vi "NFL_Setpoint_Control.vi"(8 "error in":errorcluster, 9 "3 JSA60 DX812 XQ75":dbl, 10 "3 JSA60 DX811 XQ75":dbl, 11 "SI750.lvclass in":refnum<class "SI750.lvclass">) -> (0 "error out":errorcluster, 1 "NFL Setp Grad":dbl, 2 "NFL Setpoint":dbl, 3 "SI750.lvclass out":refnum<class "SI750.lvclass">)   [LabVIEW 2022 SP3, in "SI750.lvclass"]
uses:
  SI750.lvclass
  SI750.lvclass/SI750.ctl
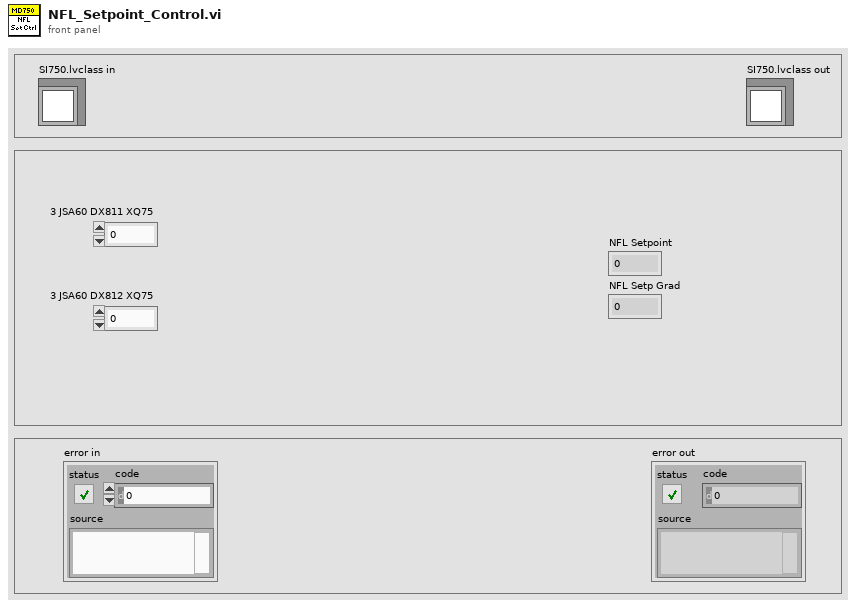
[diagram p1: front panel]
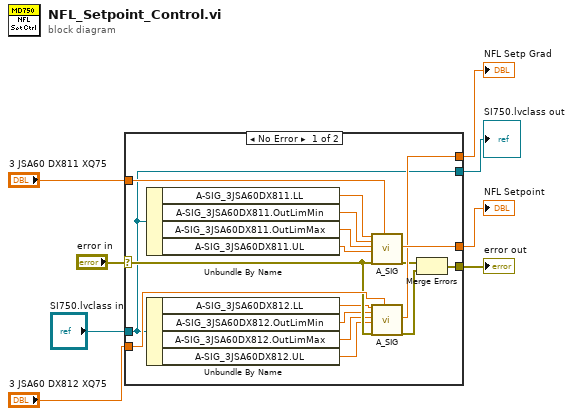
[diagram p0: block diagram]
diagram:
  n1 = case shown="No Error" "error in" {
    selector: "error in" -> [w19 w27]
    tunnel: "3 JSA60 DX811 XQ75" -> [w25 _]
    tunnel: "3 JSA60 DX812 XQ75" -> [w24 _]
    tunnel: "SI750.lvclass in" -> [w9 w26]
    tunnel: [w14 _] -> w4
    tunnel: [w13 _] -> w3
    tunnel: [w10 w27] -> w2
    tunnel: [w9 w26] -> w1
    frame No Error {
      n2 = Unbundle By Name(w9) -> ("A-SIG_3JSA60DX811.LL"=w23:dbl, "A-SIG_3JSA60DX811.OutLimMin"=w22:dbl, "A-SIG_3JSA60DX811.OutLimMax"=w21:dbl, "A-SIG_3JSA60DX811.UL"=w20:dbl)
      n3 = Unbundle By Name(w9) -> ("A-SIG_3JSA60DX812.LL"=w18:dbl, "A-SIG_3JSA60DX812.OutLimMin"=w17:dbl, "A-SIG_3JSA60DX812.OutLimMax"=w16:dbl, "A-SIG_3JSA60DX812.UL"=w15:dbl)
      n4 = call "A_SIG.vi"("LL"=w23, "OutLimMin"=w22, "OutLimMax"=w21, "UL"=w20, "error in (no error)"=w19, "Input"=w25) -> ("A_SIG_out"=w14:dbl, "error out"=w12:errorcluster)  [unwired: 12 in]
      n5 = call "A_SIG.vi"("LL"=w18, "OutLimMin"=w17, "OutLimMax"=w16, "UL"=w15, "error in (no error)"=w19, "Input"=w24) -> ("A_SIG_out"=w13:dbl, "error out"=w11:errorcluster)  [unwired: 12 in]
      n6 = Merge Errors(w12, w11) -> (w10:errorcluster)
    }
    frame Error {
    }
  }
  "NFL Setpoint" <- w4
  "NFL Setp Grad" <- w3
  "error out" <- w2
  "SI750.lvclass out" <- w1
